vi "ResonanceAnalyzer.vi"() -> ()   [LabVIEW 2015]
uses:
  <vilib>/imath/engines/lvmath2/RunTimeEngine/Managers/WorkSpace/UID Generator.vi
  <vilib>/imath/engines/lvmath2/RunTimeEngine/RangeToken/NIMS_Range.vi
  <instcachedir>/0/NIMS_Range_D919CC09935940E88F755EC1C6F49AC1.lvgen/NIMS_Range_D919CC09935940E88F755EC1C6F49AC1_000.vi
  <vilib>/imath/engines/lvmath2/RunTimeEngine/RunTimeType/NIMS_RunTimeType_From StrictType (excl LVString).vi
  <instcachedir>/0/NIMS_RunTimeType_From StrictType (excl LVString)_EB1C38A9BC5048DA9ABDA8F781E54D21.lvgen/NIMS_RunTimeType_From StrictType (excl LVString)_EB1C38A9BC5048DA9ABDA8F781E54D21_000.vi
  <vilib>/imathl/engines/lvmath/Functions/Error Handling/Create Error.vi
  <vilib>/imath/engines/lvmath2/RunTimeEngine/LocalVariableDefStatement/MC_LocalVariableDefStatement_Display.vi
  <vilib>/imath/engines/lvmath2/RunTimeEngine/ArithmeticOperatorToken/NIMS_ArithmeticOperator_minus.vi
  <instcachedir>/0/NIMS_ArithmeticOperator_minus_8228ED1EA52B4CB8A68367813E4B0C9D.lvgen/NIMS_ArithmeticOperator_minus_8228ED1EA52B4CB8A68367813E4B0C9D_003.vi
  <vilib>/imath/engines/lvmath2/RunTimeEngine/BuiltInFunctions/randnormal/NIMS_randnormal(1,I32).vi
  <vilib>/imath/engines/lvmath2/RunTimeEngine/ErrorHandling/NIMS_Error From Error Code.vi
  <vilib>/imath/engines/lvmath2/RunTimeEngine/ArithmeticOperatorToken/NIMS_ArithmeticOperator_plus.vi
  <instcachedir>/0/NIMS_ArithmeticOperator_plus_A4F2756F5ADB4A0090E0DBD7C10701C8.lvgen/NIMS_ArithmeticOperator_plus_A4F2756F5ADB4A0090E0DBD7C10701C8_000.vi
  <vilib>/imath/engines/lvmath2/RunTimeEngine/Managers/SymbolTable/Clear UID.vi
  <vilib>/imath/engines/lvmath2/RunTimeEngine/NodeEndStatement/NIMS_NodeEndStatement_Output.vi
  <instcachedir>/0/NIMS_NodeEndStatement_Output_53EC0D466D134D7ABD903AC30B43404B.lvgen/NIMS_NodeEndStatement_Output_53EC0D466D134D7ABD903AC30B43404B_000.vi
  <instcachedir>/0/NIMS_NodeEndStatement_Output_53EC0D466D134D7ABD903AC30B43404B.lvgen/NIMS_NodeEndStatement_Output_53EC0D466D134D7ABD903AC30B43404B_005.vi
  <vilib>/imath/engines/lvmath2/RunTimeEngine/ErrorHandling/NIMS_Finalize Error.vi
  <vilib>/imath/engines/lvmath2/RunTimeEngine/Managers/SymbolTable/NIMS_WorkSpace.lvlib
panel:
  out "Results":T1={"Q"=9.921370709770164, "Amplitude"=0.9962303509989965, "Center Frequency"=600.0558473917959}
  out "Resonance Curve":cluster{"all rows":dbl[], "gn":dbl[]}[](graph)=[{"all rows"=[400.0, 405.0, 410.0, 415.0, 420.0, 425.0, 430.0, 435.0, 440.0, 445.0, 450.0, 455.0, 460.0, 465.0, 470.0, 475.0, 480.0, 485.0, 490.0, 495.0, 500.0, 505.0, 510.0, 515.0, 520.0, 525.0, 530.0, 535.0, 540.0, 545.0, 550.0, 555.0, 560.0, 565.0, 570.0, 575.0, 580.0, 585.0, 590.0, 595.0, 600.0, 605.0, 610.0, 615.0, 620.0, 625.0, 630.0, 635.0, 640.0, 645.0, 650.0, 655.0, 660.0, 665.0, 670.0, 675.0, 680.0, 685.0, 690.0, 695.0, 700.0, 705.0, 710.0, 715.0, 720.0, 725.0, 730.0, 735.0, 740.0, 745.0, 750.0, 755.0, 760.0, 765.0, 770.0, 775.0, 780.0, 785.0, 790.0, 795.0, 800.0], "gn"=[0.11945794874579085, 0.13079217401378282, 0.13256380545656574, 0.1396101983493541, 0.1511386116038743, 0.1591364323537324, 0.1504717489330716, 0.161066805434556, 0.16592547069380864, 0.15528605328913073, 0.17137599536196696, 0.1749535683239119, 0.19460675733991598, 0.19301025282645323, 0.19942327889948408, 0.22009112987660134, 0.22729004652559, 0.21977225910876763, 0.22967241044761855, 0.27023571183813927, 0.27293488951083644, 0.28172005030077185, 0.310252410518223, 0.2952708672992617, 0.32561174608668875, 0.3369535596706286, 0.38017261569182453, 0.40226287654107934, 0.42501888925993825, 0.47522731133855656, 0.49600577535713736, 0.543835133840149, 0.566788438898934, 0.6337048171668601, 0.7026230928333422, 0.7566073086175669, 0.8208151602378904, 0.896818015110111, 0.9436669439605023, 0.9726262436692859, 1.0052233573630405, 0.984043218913538, 0.946866422854582, 0.8955673951255662, 0.8480140812185554, 0.7695379665051041, 0.716745476249607, 0.6589331456981307, 0.6076126465141074, 0.566878073351936, 0.5362093566452778, 0.4914063052083436, 0.4631625552626213, 0.4380401315130436, 0.42393358519077545, 0.3880730841297721, 0.36554319476699926, 0.3540746800283833, 0.3282344974936979, 0.3358141287396211, 0.294817733954048, 0.30316532199369883, 0.28680336647358995, 0.2551324150833609, 0.26237441876692025, 0.24900607841163305, 0.24372466725607503, 0.24927388618002883, 0.24155075098463788, 0.22901310072425213, 0.2090000385409277, 0.21407129077801734, 0.1774645594733686, 0.20375497812589982, 0.1996080839363432, 0.17664237920967624, 0.17891404812573825, 0.1747446562333389, 0.17297991587620604, 0.19928694230279928, 0.16833106781170204]}, {"all rows"=[400.0, 405.0, 410.0, 415.0, 420.0, 425.0, 430.0, 435.0, 440.0, 445.0, 450.0, 455.0, 460.0, 465.0, 470.0, 475.0, 480.0, 485.0, 490.0, 495.0, 500.0, 505.0, 510.0, 515.0, 520.0, 525.0, 530.0, 535.0, 540.0, 545.0, 550.0, 555.0, 560.0, 565.0, 570.0, 575.0, 580.0, 585.0, 590.0, 595.0, 600.0, 605.0, 610.0, 615.0, 620.0, 625.0, 630.0, 635.0, 640.0, 645.0, 650.0, 655.0, 660.0, 665.0, 670.0, 675.0, 680.0, 685.0, 690.0, 695.0, 700.0, 705.0, 710.0, 715.0, 720.0, 725.0, 730.0, 735.0, 740.0, 745.0, 750.0, 755.0, 760.0, 765.0, 770.0, 775.0, 780.0, 785.0, 790.0, 795.0, 800.0], "gn"=[0.11959474536814, 0.12351558479070418, 0.127627292872633, 0.13194478621964198, 0.13648453524025658, 0.14126476864264703, 0.14630571039746615, 0.15162985518592426, 0.1572622896191647, 0.16323106807585286, 0.16956765393222237, 0.1763074393427804, 0.18349035968176408, 0.19116162241101486, 0.19937257466144345, 0.2081817393902068, 0.21765605680826686, 0.22787237605996918, 0.23891925201289943, 0.25089911344333066, 0.2639308814417152, 0.2781531292404744, 0.2937278839394723, 0.3108451705751425, 0.329728377201149, 0.35064045179604614, 0.37389078114897517, 0.3998422597511346, 0.4289173672060299, 0.4616007308446504, 0.49843311306197263, 0.5399871190813724, 0.5868068235162385, 0.6392805773337118, 0.6973991858010952, 0.760340190241975, 0.8258480695045741, 0.8895289261823566, 0.9445306453368215, 0.982478703123059, 0.9962286519931356, 0.9832810982432127, 0.947127066387602, 0.8952510324048726, 0.8356994523733635, 0.7747417213349256, 0.7162783850127715, 0.6622723543553162, 0.6134245521047247, 0.5697288255631525, 0.530834622542632, 0.4962560342035444, 0.46548175250887514, 0.43802762484643826, 0.41345815114001533, 0.3913921266948442, 0.37150074621376045, 0.3535025393954241, 0.3371573437135938, 0.3222603658839483, 0.3086367838539993, 0.29613703913707395, 0.28463282441367305, 0.2740137078489752, 0.264184313214596, 0.25506197242420314, 0.24657477347414347, 0.23865993642947309, 0.23126246028538877, 0.22433399302985063, 0.21783188556291677, 0.21171839719454832, 0.2059600263198666, 0.20052694470138352, 0.19539251773013747, 0.19053289624267725, 0.18592666807169192, 0.18155455961795577, 0.17739917944396585, 0.17344479728192574, 0.16967715298267266]}]
  in  "?":enum32{"Simulation", "Experiment"}(tab)
  in  "Input Parameters":T2={"Q"=10.0, "Center Frequency"=600.0, "Start Frequency"=400.0, "End Frequency"=800.0, "df"=5.0, "Noise Level"=0.01}
  in  "Data":path
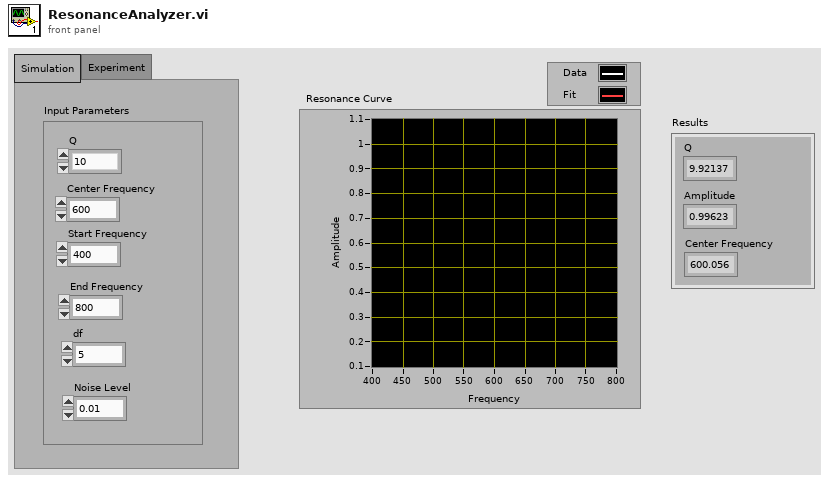
[diagram p1: front panel]
types:
  T1 = cluster{"Q":dbl, "Amplitude":dbl, "Center Frequency":dbl}
  T2 = cluster{"Q":dbl, "Center Frequency":dbl, "Start Frequency":dbl, "End Frequency":dbl, "df":dbl, "Noise Level":dbl}
  T3 = cluster{"Array[0]":dbl, "Array[1]":dbl, "Array[2]":dbl, "Array[3]":dbl, "Array[4]":dbl, "Array[5]":dbl, "Array[6]":dbl, "Array[7]":dbl, "Array[8]":dbl}
  T4 = cluster{"Array[1]":dbl, "Array[0]":dbl, "Array[2]":dbl}
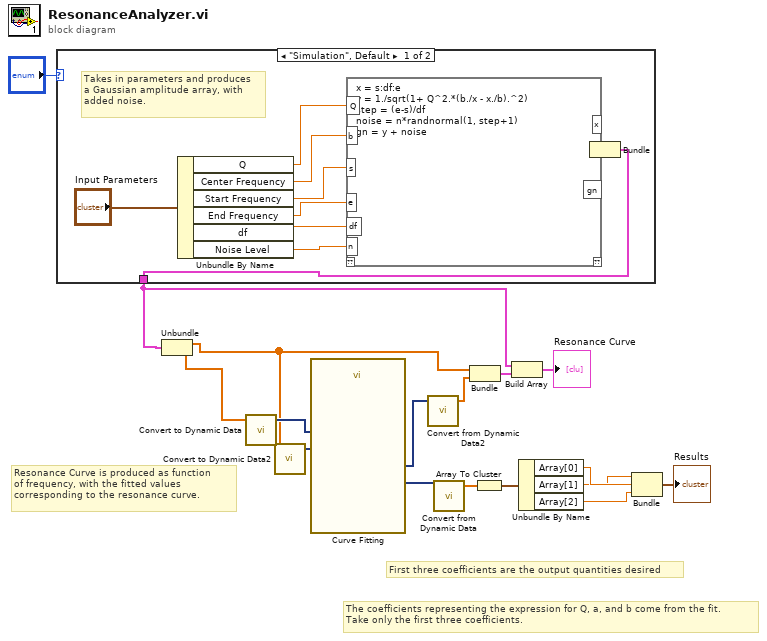
[diagram p0: block diagram]
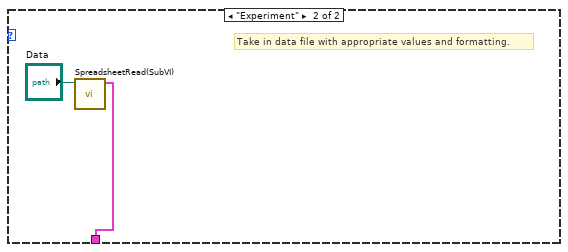
[diagram p2: hidden frame]
diagram:
  # "The coefficients representing the expression for Q, a, and b come from the fit. \nTake only the first three coefficients."
  # "Resonance Curve is produced as function \nof frequency, with the fitted values\ncorresponding to the resonance curve."
  # "First three coefficients are the output quantities desired"
  n1 = case shown="\"Simulation\", Default" "?" {
    tunnel: [w18 w198] -> w5
    frame "Simulation", Default {
      # "Takes in parameters and produces\na Gaussian amplitude array, with\nadded noise."
      n2 = Unbundle By Name("Input Parameters") -> ("Q"=w26:dbl, "Center Frequency"=w25:dbl, "Start Frequency"=w24:dbl, "End Frequency"=w23:dbl, "df"=w22:dbl, "Noise Level"=w21:dbl)
      n3 = mathscript code="x = s:df:e\ny = 1./sqrt(1+ Q^2.*(b./x - x./b).^2)\nstep = (e-s)/df\nnoise = n*randnormal(1, step+1)\ngn = y + noise"("Q"=w26, "b"=w25, "s"=w24, "e"=w23, "df"=w22, "n"=w21) -> ("x"=w19:dbl[], "gn"=w20:cdb[])  [unwired: 1 in, 1 out]
      n4 = Bundle("x"=w19, "gn"=w20) -> (w18:cluster{"x":dbl[], "gn":cdb[]})  [unwired: 1 in]
    }
    frame "Experiment" {
      # "Take in data file with appropriate values and formatting."
      n5 = call "SpreadsheetRead(SubVI).vi"("Path"="Data") -> ("Cluster"=w198:cluster{"all rows":dbl[], "all rows":dbl[]})  [unwired: 10 in]
    }
  }
  n6 = Unbundle(w5) -> ("all rows"=w4:dbl[], "gn"=w3:cdb[])
  n7 = call "Convert to Dynamic Data"("Array"=w3) -> ("Dynamic Data Type"=w10:dynamicdata)  [unwired: 3 in]
  n8 = call "Convert to Dynamic Data2"("Array"=w4) -> ("Dynamic Data Type"=w6:dynamicdata)  [unwired: 3 in]
  n9 = call "Curve Fitting"("Locations"=w6, "Signals"=w10) -> ("best fit"=w9:dynamicdata, "non-linear coefficients"=w11:dynamicdata)  [unwired: 5 in, 3 out]
  n10 = call "Convert from Dynamic Data2"("Dynamic Data Type"=w9) -> ("Array"=w8:dbl[])  [unwired: 3 in]
  n11 = call "Convert from Dynamic Data"("Dynamic Data Type"=w11) -> ("Array"=w17:dbl[])  [unwired: 3 in]
  n12 = Bundle("all rows"=w4, "Array"=w8) -> (w7:cluster{"all rows":dbl[], "Array":dbl[]})  [unwired: 1 in]
  n13 = Array To Cluster(array=w17) -> (cluster=w15:T3)
  n14 = Build Array(w5, w7) -> (→"Resonance Curve":cluster{"all rows":dbl[], "gn":cdb[]}[])
  n15 = Unbundle By Name(w15) -> ("Array[0]"=w2:dbl, "Array[1]"=w1:dbl, "Array[2]"=w14:dbl)
  n16 = Bundle("Array[1]"=w1, "Array[0]"=w2, "Array[2]"=w14) -> (→"Results":T4)  [unwired: 1 in]
